vi "Set Identity.vi"(8 "error in (no error)":errorcluster, 9 "Name(\"\")":string, 10 "ID(\"\")":string, 11 "MemberInfo in":refnum<class "Information.lvclass">) -> (0 "error out":errorcluster, 3 "MemberInfo out":refnum<class "Information.lvclass">)   [LabVIEW 2015, in "Information.lvclass"]
uses:
  Information.lvclass
  Information.lvclass/Information.ctl
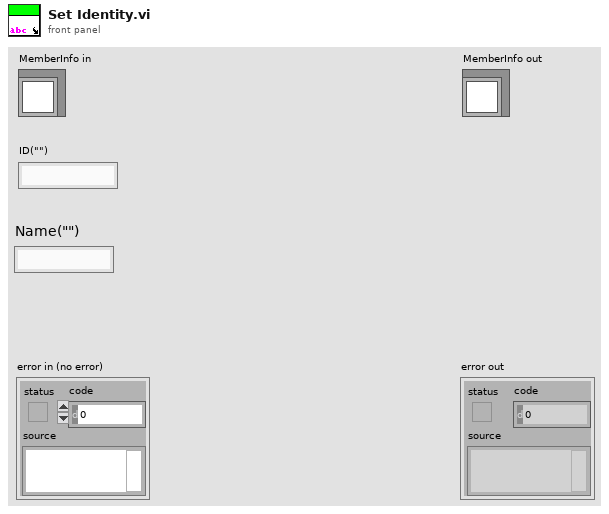
[diagram p1: front panel]
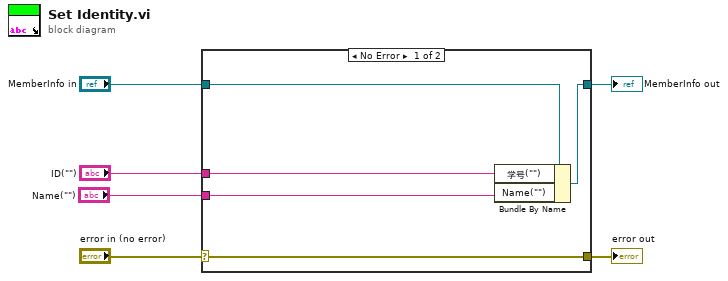
[diagram p0: block diagram]
diagram:
  n1 = case shown="No Error" "error in (no error)" {
    selector: "error in (no error)" -> [w11 w12]
    tunnel: [w11 w12] -> w5
    tunnel: [w9 w13] -> w3
    tunnel: "MemberInfo in" -> [w10 w13]
    tunnel: "ID(\"\")" -> [w8 _]
    tunnel: "Name(\"\")" -> [w7 _]
    frame No Error {
      n2 = Bundle By Name(cluster=w10, "学号(\"\")"=w8, "Name(\"\")"=w7) -> (w9:refnum<class "Information.lvclass">)
    }
    frame Error {
    }
  }
  "error out" <- w5
  "MemberInfo out" <- w3
